vi "Clear Empty Parents.vi"(8 "error in (no error)":errorcluster, 11 "TreeControl in":refnum<vi>) -> (0 "error IO":errorcluster)   [LabVIEW 2020]
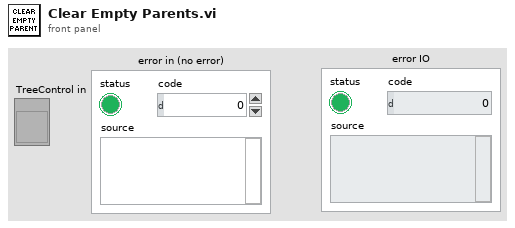
[diagram p1: front panel]
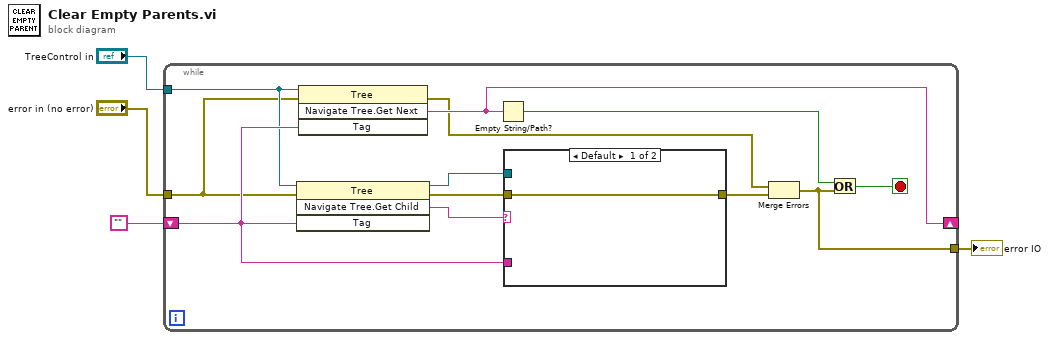
[diagram p0: block diagram]
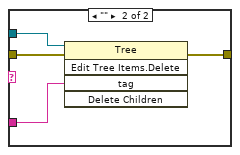
[diagram p2: hidden frame]
diagram:
  n1 = while {
    tunnel: "TreeControl in" -> [w11]
    shift-right: [w12] -> _
    shift-left: "" -> [w14]
    tunnel: "error in (no error)" -> [w10]
    tunnel: [w5] -> w1
    stop <- w8 stop-if-true
    n2 = invoke class="Tree" method="Navigate Tree.Get Child"(reference=w11, error in=w10, "Tag"=w14) -> (reference out=w15:refnum<vi>, error out=w9:errorcluster, "Navigate Tree:Get Child"=w16:string)  [unwired: 1 in, 1 out]
    n3 = invoke class="Tree" method="Navigate Tree.Get Next"(reference=w11, error in=w10, "Tag"=w14) -> (error out=w6:errorcluster, "Navigate Tree:Get Next Item"=w12:string)  [unwired: 1 in, 2 out]
    n4 = Empty String/Path?(string/path=w12) -> (empty?=w13:bool)
    n5 = case shown="Default" w16 {
      tunnel: w15 -> [_ w21]
      tunnel: w14 -> [_ w20]
      tunnel: w9 -> [w17 w19]
      tunnel: [w17 w18] -> w7
      frame Default {
      }
      frame "" {
        n6 = invoke class="Tree" method="Edit Tree Items.Delete"(reference=w21, error in=w19, "tag"=w20) -> (error out=w18:errorcluster)  [unwired: 2 in, 4 out]
      }
    }
    n7 = Merge Errors(w6, w7) -> (w5:errorcluster)
    n8 = Or(x=w13, y=w5) -> (x .or. y?=w8:bool)
  }
  "error IO" <- w1
